vi "Save&ReadToText.vi"() -> ()   [LabVIEW 2018]
panel:
  in  "Array 2":variant[](array[variant])
  in  "Array":string[](array[string])
  in  "file path (use dialog)":path
  out "value":T1
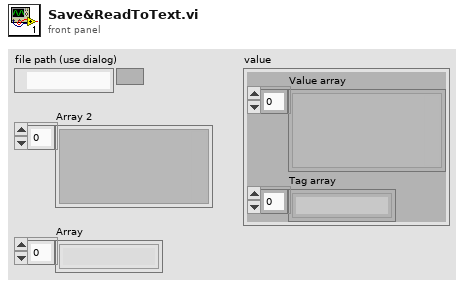
[diagram p1: front panel]
types:
  T1 = cluster{"Value array":variant[], "Tag array":string[]}
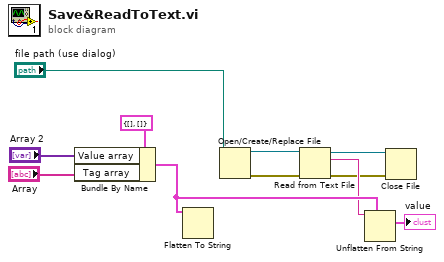
[diagram p0: block diagram]
diagram:
  n1 = Bundle By Name(cluster=T1 {"Value array"=[], "Tag array"=[]} ("input cluster"), "Value array"="Array 2", "Tag array"="Array") -> (w10:T1)
  n2 = Flatten To String(anything=w10) -> ()  [unwired: 3 in, 3 out]
  n3 = Open/Create/Replace File(file path (use dialog)="file path (use dialog)") -> (refnum out=w5:refnum<file>, error out=w6:errorcluster)  [unwired: 5 in, 1 out]
  n4 = Read from Text File(file (use dialog)=w5, error in=w6) -> (refnum out=w7:refnum<file>, text=w9:string, error out=w8:errorcluster)  [unwired: 2 in, 1 out]
  n5 = Unflatten From String(type=w10, binary string=w9) -> (value=→"value":T1)  [unwired: 3 in, 2 out]
  n6 = Close File(refnum=w7, error in=w8) -> ()  [unwired: 2 out]
